vi "video.free.vi"(8 "error in":errorcluster, 11 "Video":refnum<class "Video.lvclass">) -> (0 "error out":errorcluster)   [LabVIEW 2020, in "Video.lvclass"]
doc: "Releases the handle and its associated resources."
uses:
  Video.lvclass
  Video.lvclass/Video.ctl
  client.lvlib
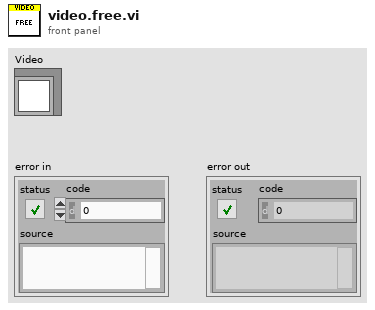
[diagram p1: front panel]
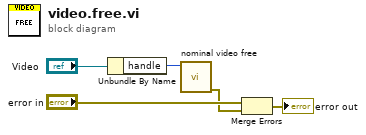
[diagram p0: block diagram]
diagram:
  n1 = Unbundle By Name("Video") -> ("handle"=w5:i32)
  n2 = call "nominal video free.vi"("video"=w5) -> ("error out"=w2:errorcluster)  [unwired: 9 in, 1 out]
  n3 = Merge Errors("error in", w2) -> (→"error out":errorcluster)
